vi "Calculate Initial Flashes.vi"(11 "Octopus Energy Matrix In":i32[][](array[numeric])) -> (0 "Flash Count":i32, 1 "Flashes Columns":i32[](array[numeric]), 2 "Flashes Rows":i32[](array[numeric]), 3 "Octopus Energy Matrix Out":i32[][](array[numeric]))   [LabVIEW 2019, in "Day 11.lvlib"]
uses:
  Day 11.lvlib
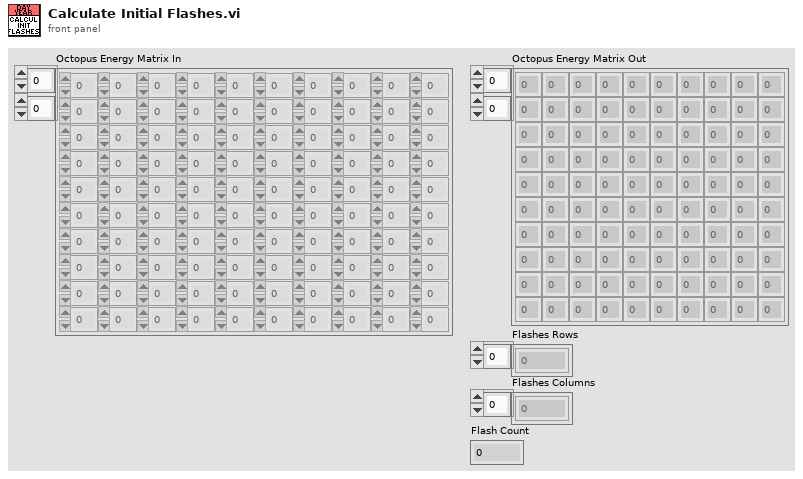
[diagram p1: front panel]
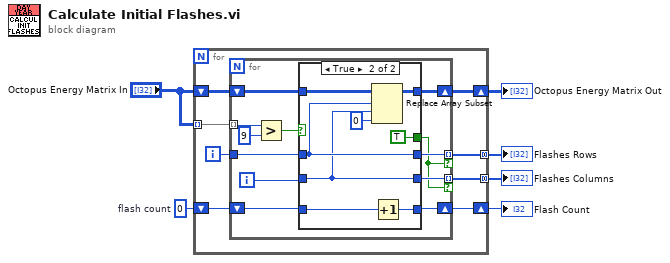
[diagram p0: block diagram]
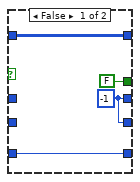
[diagram p2: hidden frame]
diagram:
  w6 = 0  # flash count
  n1 = for {
    tunnel: "Octopus Energy Matrix In" -> [w14] mode=indexing
    shift-right: [w11] -> w4
    shift-left: "Octopus Energy Matrix In" -> [w13]
    shift-right: [w9] -> w1
    shift-left: w6 -> [w10]
    tunnel: [w8] -> w3 mode=concatenating
    tunnel: [w7] -> w2 mode=concatenating
    i -> [w12]
    n2 = for {
      tunnel: w14 -> [w26] mode=indexing
      tunnel: w12 -> [w20]
      shift-right: [w23] -> w11
      shift-left: w13 -> [w24]
      shift-right: [w21] -> w9
      shift-left: w10 -> [w22]
      tunnel: [w17] -> w8 mode=indexing if=w15
      tunnel: [w16] -> w7 mode=indexing if=w15
      i -> [w19]
      n3 = Greater?(x=w26, y=9) -> (0:w18:bool)
      n4 = case shown="True" w18 {
        tunnel: w24 -> [w30 w38]
        tunnel: [w30 w36] -> w23
        tunnel: w22 -> [w28 w35]
        tunnel: [w28 w34] -> w21
        tunnel: w20 -> [_ w33]
        tunnel: w19 -> [_ w32]
        tunnel: [w29 w33] -> w17
        tunnel: [w29 w32] -> w16
        tunnel: [FALSE TRUE] -> w15
        frame False {
          w29 = -1
        }
        frame True {
          n5 = Replace Array Subset(array=w38, new element=0 ("new element/subarray"), index (row)=w33, index (col)=w32) -> (w36:i32[][])
          n6 = Increment(x=w35) -> (x+1=w34:i32)
        }
      }
    }
  }
  "Octopus Energy Matrix Out" <- w4
  "Flashes Rows" <- w3
  "Flashes Columns" <- w2
  "Flash Count" <- w1
